vi "conv.symbol.vi"(11 "symbol.in":string) -> (3 "symbol.out":u64 format="%.0x")   [LabVIEW 2020, in "fpganow.common.host.lvlib"]
uses:
  fpganow.common.host.lvlib
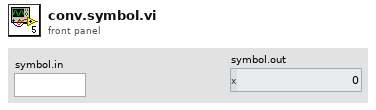
[diagram p1: front panel]
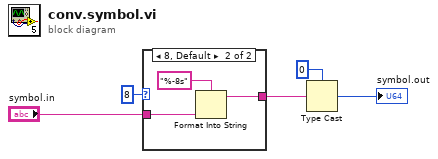
[diagram p0: block diagram]
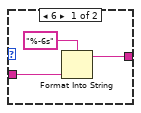
[diagram p2: hidden frame]
diagram:
  n1 = case shown="8, Default" 8 ("Length") {
    tunnel: [w8 w11] -> w3
    tunnel: "symbol.in" -> [w6 w9]
    frame 6 {
      n2 = Format Into String(format string="%-6s", w6) -> (resulting string=w8:string)  [unwired: 2 in, 1 out]
    }
    frame 8, Default {
      n3 = Format Into String(format string="%-8s", w9) -> (resulting string=w11:string)  [unwired: 2 in, 1 out]
    }
  }
  n4 = Type Cast(type=u64 0, x=w3) -> (*(type *) &x=→"symbol.out":u64)
